vi "Sandbox4.vi"() -> ()   [LabVIEW 2014]
panel:
  in  "Tree":string(tree)
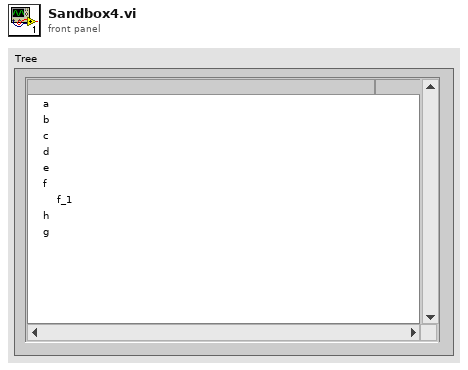
[diagram p1: front panel]
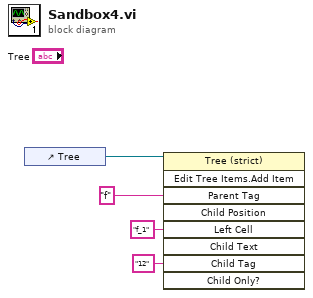
[diagram p0: block diagram]
diagram:
  n1 = control-ref of="Tree"() -> (w4:refnum<vi>)
  n2 = invoke class="Tree (strict)" method="Edit Tree Items.Add Item"(reference=w4, "Parent Tag"="f", "Left Cell"="f_1" ("Left Cell String"), "Child Tag"="12") -> ()  [unwired: 5 in, 9 out]
